vi "Main Host Json Commands.vi"(8 "error in":errorcluster, 10 "main queue":refnum<queue>, 11 "tcp in":refnum<k5>) -> (0 "error out":errorcluster, 2 "processed?":bool, 3 "tcp out":refnum<k5>)   [LabVIEW 2019]
uses:
  <vilib>/Utility/error.llb/DialogType.ctl
  RT Controls/Main Command Events.ctl
  RT Controls/Main Process Commands.ctl
panel:
  out "full cmd":string
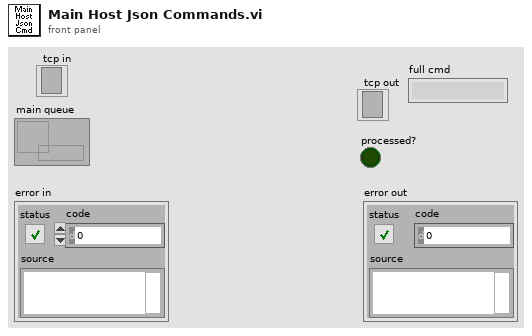
[diagram p1: front panel]
types:
  T1 = enum16{"Standard", "Buffered", "CRLF", "Immediate"}
  T2 = typedef "DialogType.ctl" = u16
  T3 = typedef "Main Process Commands.ctl" = cluster{"Commands":T4, "Value":variant}
  T4 = typedef "Main Command Events.ctl" = enum16{"Idle", "FullStop", "MainReadConfig", "MainWriteConfig", "OpenUpper", "CloseUpper", "OpenLower", "CloseLower", "SetWatchdogInt", "EnRainShutDn", "DisRainShutDn", "EnCloudShutDn", "DisCloudShutDn", "SetRainDelay", "SetLowerTimLim", "EnAutoShutDn", "DisAutoShutDn", "SetRevDelay", "RotToAz", "RotLeft", "RotRight", "RotToHome", "DefineHomePos", "SetCoast", "SetHSThres", "SetEncCounts", "SyncClose", "SyncOpen", "SetAZTimLim", "SetHomeEncPos", "SetAZTol", "SetDoorMoveTO", "AZEncPositive", "AZEncNegative", "SetShutdown", "RotToCenter"}
  T5 = cluster{"reply":string, "value":string, "error":errorcluster}
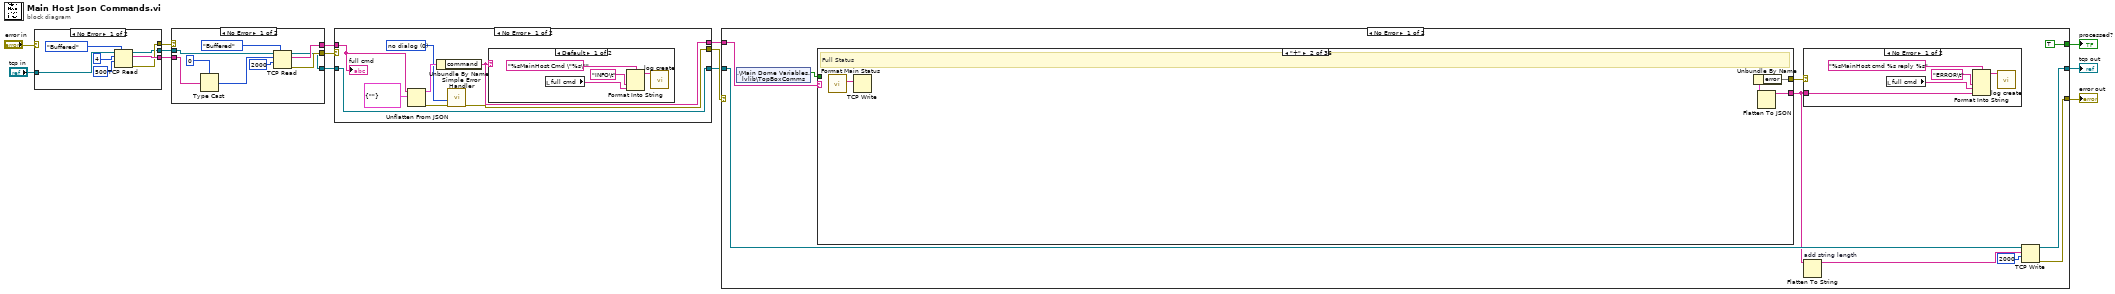
[diagram p0: block diagram]
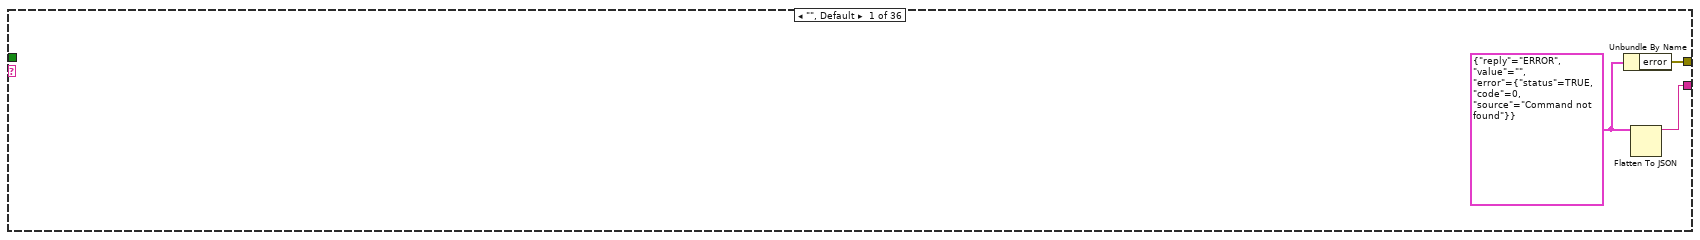
[diagram p3: hidden frame]
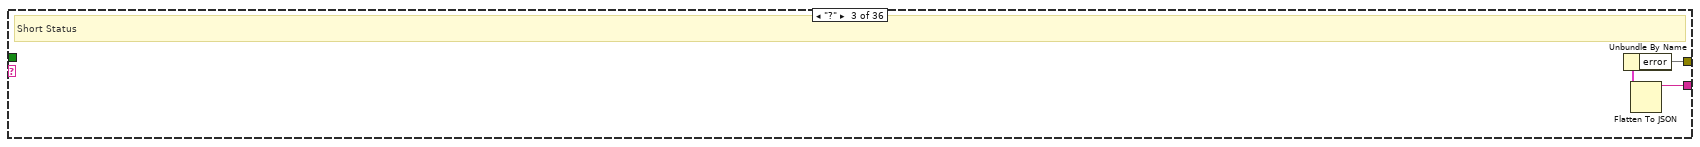
[diagram p4: hidden frame]
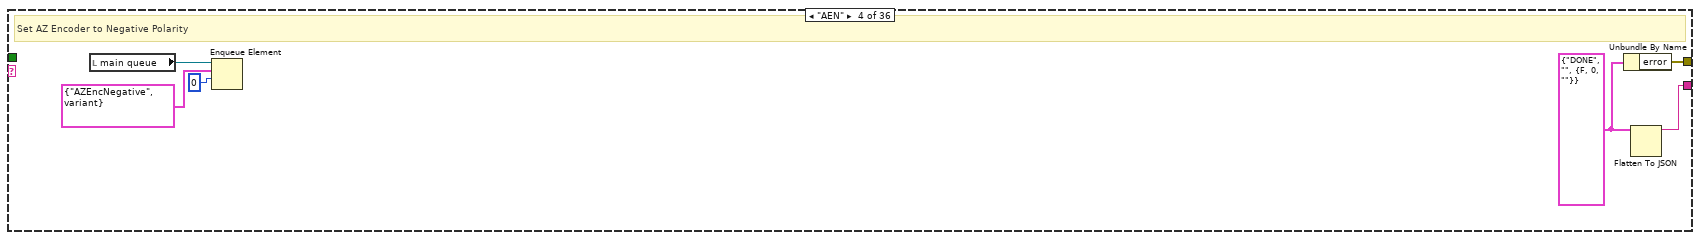
[diagram p5: hidden frame]
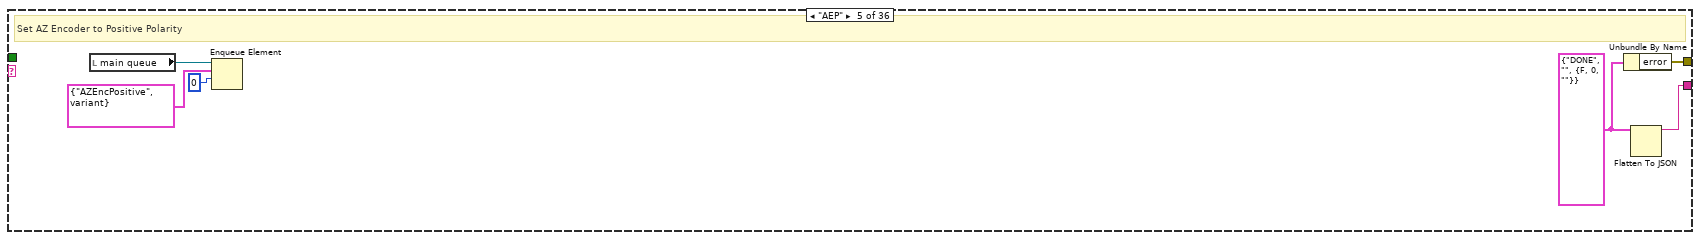
[diagram p6: hidden frame]
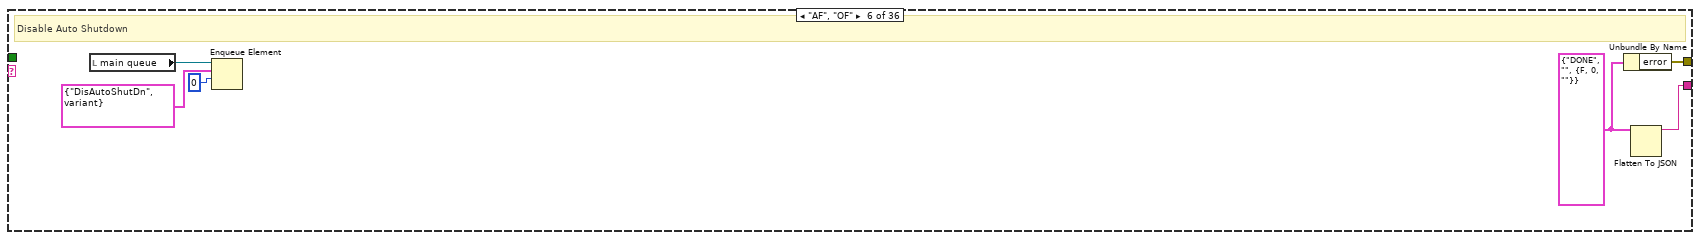
[diagram p7: hidden frame]
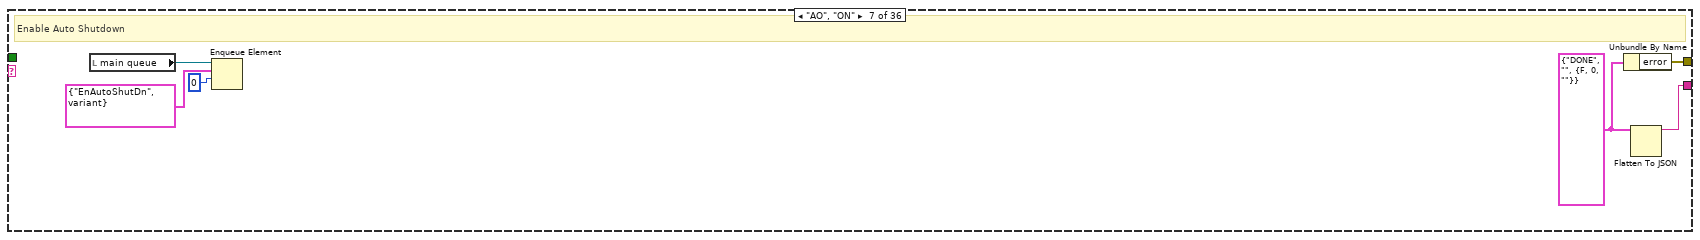
[diagram p8: hidden frame]
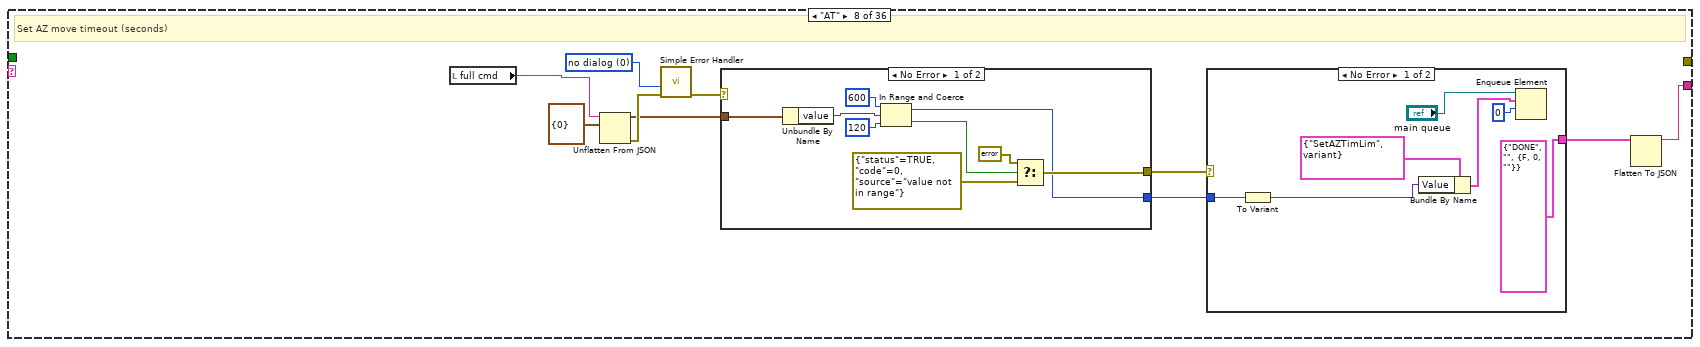
[diagram p9: hidden frame]
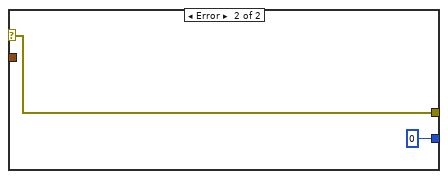
[diagram p10: hidden frame]
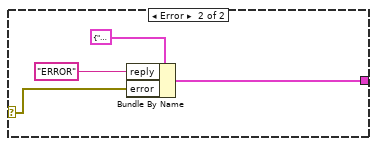
[diagram p11: hidden frame]
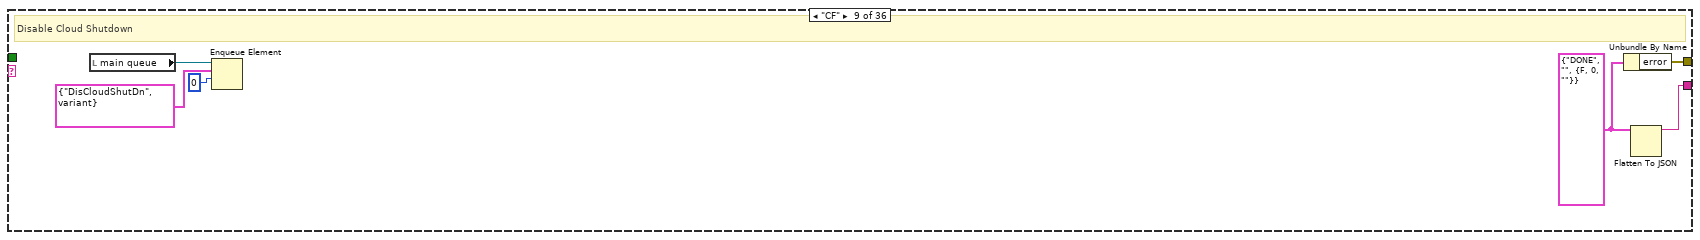
[diagram p12: hidden frame]
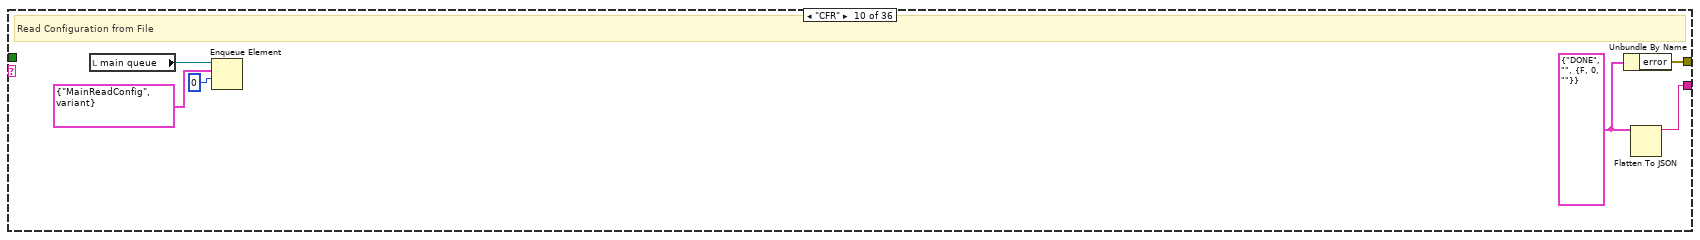
[diagram p13: hidden frame]
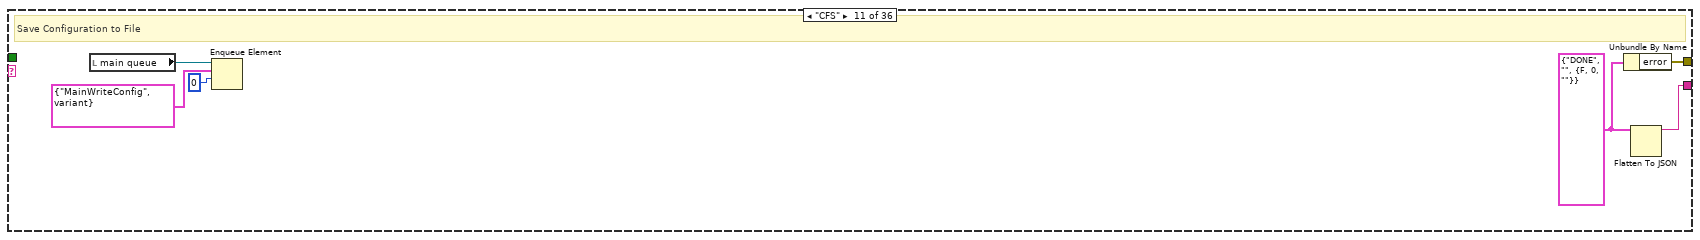
[diagram p14: hidden frame]
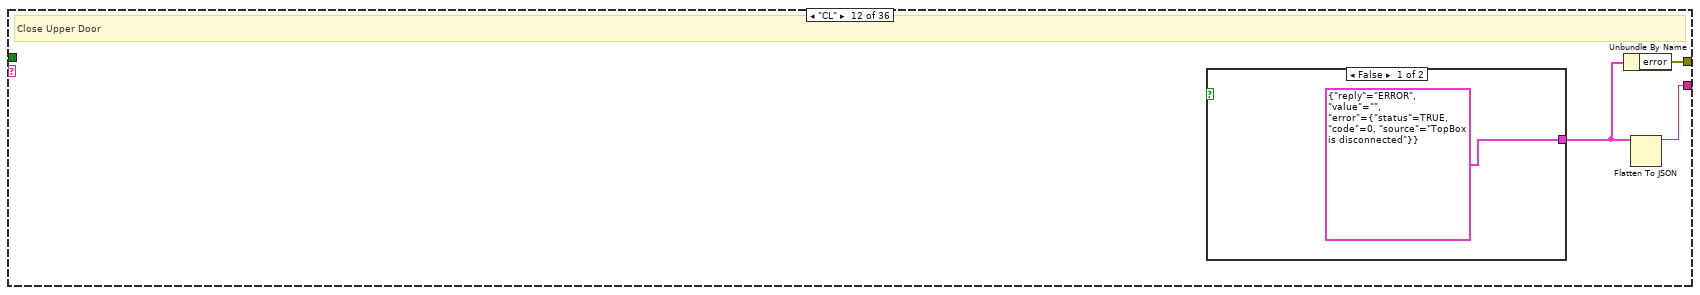
[diagram p15: hidden frame]
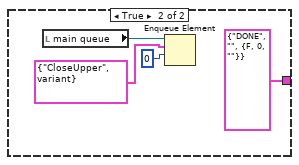
[diagram p16: hidden frame]
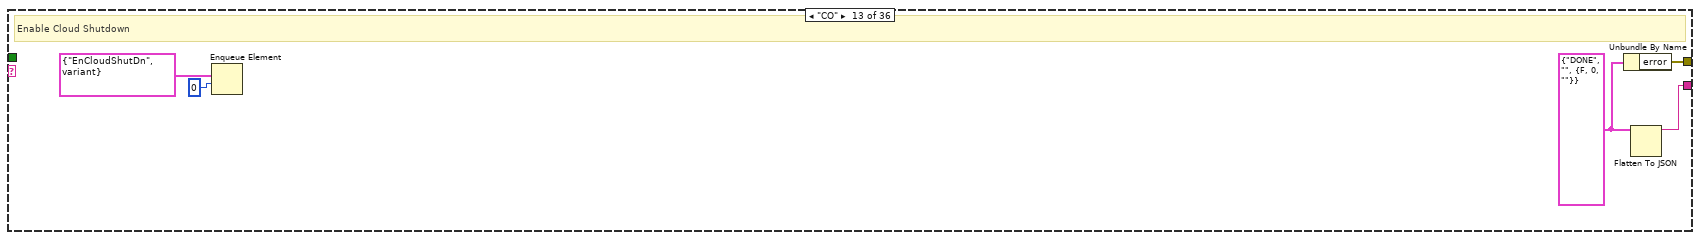
[diagram p17: hidden frame]
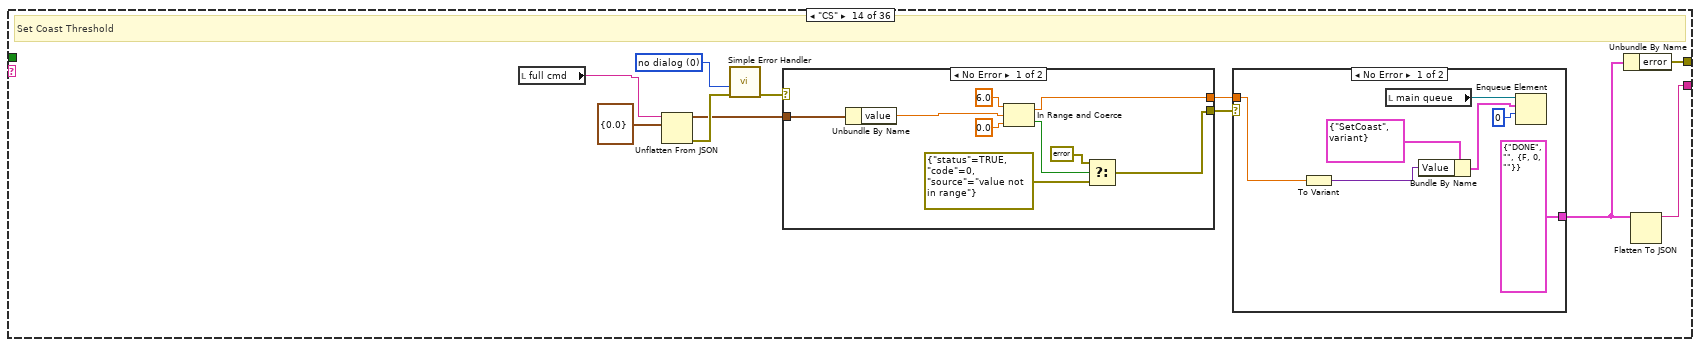
[diagram p18: hidden frame]
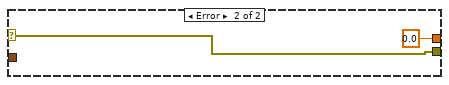
[diagram p19: hidden frame]
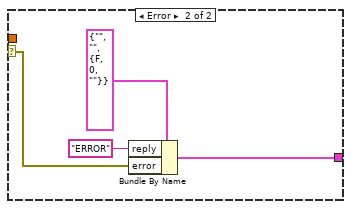
[diagram p20: hidden frame]
diagram:
  n1 = case shown="No Error" "error in" {
    selector: "error in" -> [_ w24]
    tunnel: "tcp in" -> [w21 w22]
    tunnel: [w17 "" ("data out")] -> w12
    tunnel: [w16 w24] -> w11
    tunnel: [w15 w22] -> w10
    frame No Error {
      n2 = TCP Read(connection ID=w21, bytes to read=4, 7:T1."Buffered" ("mode (standard)"), 9:500 ("timeout ms (25000)")) -> (connection ID out=w15:refnum<k5>, data out=w17:string, error out=w16:errorcluster)  [unwired: 1 in]
    }
    frame Error {
    }
  }
  n3 = case shown="No Error" w11 {
    selector: w11 -> [_ w34]
    tunnel: w12 -> [w33 _]
    tunnel: w10 -> [w31 w36]
    tunnel: [w28 w34] -> w9
    tunnel: [w27 "" ("data out")] -> w8
    tunnel: [w25 w36] -> w7
    frame No Error {
      n4 = Type Cast(type=0 ("length"), x=w33) -> (*(type *) &x=w30:i32)
      n5 = TCP Read(connection ID=w31, bytes to read=w30, 7:T1."Buffered" ("mode (standard)"), 9:2000 ("timeout ms (25000)")) -> (connection ID out=w25:refnum<k5>, data out=w27:string, error out=w28:errorcluster)  [unwired: 1 in]
    }
    frame Error {
    }
  }
  n6 = case shown="No Error" w9 {
    selector: w9 -> [_ w52]
    tunnel: w8 -> [w44 _]
    tunnel: w7 -> [w38 w51]
    tunnel: [w38 w51] -> w4
    tunnel: [w39 w50] -> w6
    tunnel: [w37 "" ("command")] -> w5
    frame No Error {
      w40 = T2 0 items=["no dialog", "OK message", "continue or stop message", "OK message + warnings", "continue/stop + warnings"] ("type of dialog (OK msg:1)")
      n7 = Unflatten From JSON(JSON string=w44, type and defaults=cluster{"command":string} {"command"=""}) -> (value=w42:cluster{"command":string}, error out=w41:errorcluster)  [unwired: 5 in]
      n8 = Unbundle By Name(w42) -> ("command"=w37:string)
      n9 = call <vilib>:"Simple Error Handler.vi"("type of dialog (OK msg:1)"=w40, "error in (no error)"=w41) -> ("error out"=w39:errorcluster)  [unwired: 3 in, 4 out]
      n10 = case shown="Default" w37 {
        frame Default {
          n11 = local read "full cmd"() -> (w45:string)
          n12 = Format Into String(format string="%sMainHost Cmd \"%s\"", "INFO\t" ("input 1"), w45) -> (resulting string=w46:string)  [unwired: 2 in, 1 out]
          n13 = call "log create.vi"("message"=w46) -> ()  [unwired: 11 in]
        }
        frame "+", "?", "HELP" {
        }
      }
      "full cmd" <- w44
    }
    frame Error {
      n14 = call <vilib>:"Clear Errors.vi"("error in (no error)"=w52, "specific error code to clear (0: all)"=56) -> ("error out"=w50:errorcluster)  [unwired: 4 in, 1 out]
    }
  }
  n15 = case shown="No Error" w6 {
    selector: w6 -> [_ w636]
    tunnel: w5 -> [w63 _]
    tunnel: w4 -> [w62 w634]
    tunnel: [w56 w636] -> w2
    tunnel: [TRUE FALSE] -> w3
    tunnel: [w58 w634] -> w1
    frame No Error {
      n16 = shared-variable ".\\Main Dome Variables.lvlib\\TopBoxComms"() -> (w54:bool)  [unwired: 1 in, 1 out]
      n17 = case shown="\"+\"" w63 {
        tunnel: [w71 w72 w76 w80 w87 w93 w99 w103 w137 w143 w149 w153 w162 w168 w202 w215 w248 w252 w257 w271 w304 w337 w368 w391 w416 w433 w458 w467 w484 w517 w542 w551 w560 w573 w598 w615] -> w59
        tunnel: [w69 w73 w77 w82 w86 w92 w98 _ w136 w142 w148 w155 w161 w166 w200 w216 w249 w251 w256 w272 w305 w338 w369 w392 w417 w434 w459 w468 w485 w518 w543 w552 w559 w574 w599 w616] -> w60
        tunnel: w54 -> [_ _ _ _ _ _ _ _ _ _ _ _ _ _ w199 w208 _ _ _ _ _ _ _ _ w415 _ w457 w466 _ _ w541 w550 _ _ w597 _]
        frame "", Default {
          w70 = T5 {"reply"="ERROR", "value"="", "error"={"status"=TRUE, "code"=0, "source"="Command not found"}} ("output cluster")
          n18 = Unbundle By Name(w70) -> ("error"=w69:errorcluster)
          n19 = Flatten To JSON(anything=w70) -> (JSON string=w71:string)  [unwired: 2 in, 1 out]
        }
        frame "+" {
          # "Full Status"
          n20 = call "Format Main Status.vi"() -> ("FullStat"=w75:string)  [unwired: 10 in, 1 out]
          n21 = TCP Write(data in=w75) -> ()  [unwired: 3 in, 3 out]
          n22 = Flatten To JSON() -> (anything=w74:cluster{}, JSON string=w72:string)  [unwired: 2 in, 1 out]
          n23 = Unbundle By Name(w74) -> ("error"=w73)
        }
        frame "?" {
          # "Short Status"
          n24 = Flatten To JSON() -> (anything=w78:cluster{}, JSON string=w76:string)  [unwired: 2 in, 1 out]
          n25 = Unbundle By Name(w78) -> ("error"=w77)
        }
        frame "AEN" {
          w81 = T5 {"reply"="DONE", "value"="", "error"={"status"=FALSE, "code"=0, "source"=""}} ("output cluster")
          # "Set AZ Encoder to Negative Polarity"
          n26 = local read "main queue"() -> (w79:refnum<queue>)
          n27 = Enqueue Element(queue=w79, element=T3 {"Commands"=enum."AZEncNegative", "Value"=variant} ("event data"), timeout in ms (-1)=0) -> ()  [unwired: 1 in, 3 out]
          n28 = Unbundle By Name(w81) -> ("error"=w82:errorcluster)
          n29 = Flatten To JSON(anything=w81) -> (JSON string=w80:string)  [unwired: 2 in, 1 out]
        }
        frame "AEP" {
          w88 = T5 {"reply"="DONE", "value"="", "error"={"status"=FALSE, "code"=0, "source"=""}} ("output cluster")
          # "Set AZ Encoder to Positive Polarity"
          n30 = local read "main queue"() -> (w85:refnum<queue>)
          n31 = Enqueue Element(queue=w85, element=T3 {"Commands"=enum."AZEncPositive", "Value"=variant} ("event data"), timeout in ms (-1)=0) -> ()  [unwired: 1 in, 3 out]
          n32 = Unbundle By Name(w88) -> ("error"=w86:errorcluster)
          n33 = Flatten To JSON(anything=w88) -> (JSON string=w87:string)  [unwired: 2 in, 1 out]
        }
        frame "AF", "OF" {
          w94 = T5 {"reply"="DONE", "value"="", "error"={"status"=FALSE, "code"=0, "source"=""}} ("output cluster")
          # "Disable Auto Shutdown"
          n34 = local read "main queue"() -> (w91:refnum<queue>)
          n35 = Enqueue Element(queue=w91, element=T3 {"Commands"=enum."DisAutoShutDn", "Value"=variant} ("event data"), timeout in ms (-1)=0) -> ()  [unwired: 1 in, 3 out]
          n36 = Unbundle By Name(w94) -> ("error"=w92:errorcluster)
          n37 = Flatten To JSON(anything=w94) -> (JSON string=w93:string)  [unwired: 2 in, 1 out]
        }
        frame "AO", "ON" {
          w100 = T5 {"reply"="DONE", "value"="", "error"={"status"=FALSE, "code"=0, "source"=""}} ("output cluster")
          # "Enable Auto Shutdown"
          n38 = local read "main queue"() -> (w97:refnum<queue>)
          n39 = Enqueue Element(queue=w97, element=T3 {"Commands"=enum."EnAutoShutDn", "Value"=variant} ("event data"), timeout in ms (-1)=0) -> ()  [unwired: 1 in, 3 out]
          n40 = Unbundle By Name(w100) -> ("error"=w98:errorcluster)
          n41 = Flatten To JSON(anything=w100) -> (JSON string=w99:string)  [unwired: 2 in, 1 out]
        }
        frame "AT" {
          w109 = T2 0 items=["no dialog", "OK message", "continue or stop message", "OK message + warnings", "continue/stop + warnings"] ("type of dialog (OK msg:1)")
          # "Set AZ move timeout (seconds)"
          n42 = local read "full cmd"() -> (w111:string)
          n43 = Unflatten From JSON(JSON string=w111, type and defaults=cluster{"value":i32} {"value"=0}) -> (value=w107:cluster{"value":i32}, error out=w110:errorcluster)  [unwired: 5 in]
          n44 = call <vilib>:"Simple Error Handler.vi"("type of dialog (OK msg:1)"=w109, "error in (no error)"=w110) -> ("error out"=w108:errorcluster)  [unwired: 3 in, 4 out]
          n45 = case shown="No Error" w108 {
            selector: w108 -> [_ w123]
            tunnel: w107 -> [w121 _]
            tunnel: [w115 w123] -> w106
            tunnel: [w113 0 ("upper limit")] -> w105
            frame No Error {
              n46 = Unbundle By Name(w121) -> ("value"=w118:i32)
              n47 = In Range and Coerce(upper limit=600, x=w118, lower limit=120) -> (coerced(x)=w113:i32, In Range?=w117:bool)
              n48 = Select(t=errorcluster {"status"=FALSE, "code"=0, "source"=""} ("error IO"), s=w117, f=errorcluster {"status"=TRUE, "code"=0, "source"="value not in range"}) -> (s? t:f=w115:errorcluster)
            }
            frame Error {
            }
          }
          n49 = case shown="No Error" w106 {
            selector: w106 -> [_ w133]
            tunnel: w105 -> [w130 _]
            tunnel: [T5 {"reply"="DONE", "value"="", "error"={"status"=FALSE, "code"=0, "source"=""}} ("output cluster") w132] -> w104
            frame No Error {
              n50 = To Variant(anything=w130) -> (Variant=w129:variant)
              n51 = Bundle By Name(cluster=T3 {"Commands"=enum."SetAZTimLim", "Value"=variant} ("event data"), "Value"=w129) -> (w126:T3)
              n52 = Enqueue Element(queue="main queue", element=w126, timeout in ms (-1)=0) -> ()  [unwired: 1 in, 3 out]
            }
            frame Error {
              n53 = Bundle By Name(cluster=T5 {"reply"="", "value"="", "error"={"status"=FALSE, "code"=0, "source"=""}} ("output cluster"), "reply"="ERROR", "error"=w133) -> (w132:T5)
            }
          }
          n54 = Flatten To JSON(anything=w104) -> (JSON string=w103:string)  [unwired: 2 in, 1 out]
        }
        frame "CF" {
          w138 = T5 {"reply"="DONE", "value"="", "error"={"status"=FALSE, "code"=0, "source"=""}} ("output cluster")
          # "Disable Cloud Shutdown"
          n55 = local read "main queue"() -> (w135:refnum<queue>)
          n56 = Enqueue Element(queue=w135, element=T3 {"Commands"=enum."DisCloudShutDn", "Value"=variant} ("event data"), timeout in ms (-1)=0) -> ()  [unwired: 1 in, 3 out]
          n57 = Unbundle By Name(w138) -> ("error"=w136:errorcluster)
          n58 = Flatten To JSON(anything=w138) -> (JSON string=w137:string)  [unwired: 2 in, 1 out]
        }
        frame "CFR" {
          w144 = T5 {"reply"="DONE", "value"="", "error"={"status"=FALSE, "code"=0, "source"=""}} ("output cluster")
          # "Read Configuration from File"
          n59 = local read "main queue"() -> (w141:refnum<queue>)
          n60 = Enqueue Element(queue=w141, element=T3 {"Commands"=enum."MainReadConfig", "Value"=variant} ("event data"), timeout in ms (-1)=0) -> ()  [unwired: 1 in, 3 out]
          n61 = Unbundle By Name(w144) -> ("error"=w142:errorcluster)
          n62 = Flatten To JSON(anything=w144) -> (JSON string=w143:string)  [unwired: 2 in, 1 out]
        }
        frame "CFS" {
          w150 = T5 {"reply"="DONE", "value"="", "error"={"status"=FALSE, "code"=0, "source"=""}} ("output cluster")
          # "Save Configuration to File"
          n63 = local read "main queue"() -> (w147:refnum<queue>)
          n64 = Enqueue Element(queue=w147, element=T3 {"Commands"=enum."MainWriteConfig", "Value"=variant} ("event data"), timeout in ms (-1)=0) -> ()  [unwired: 1 in, 3 out]
          n65 = Unbundle By Name(w150) -> ("error"=w148:errorcluster)
          n66 = Flatten To JSON(anything=w150) -> (JSON string=w149:string)  [unwired: 2 in, 1 out]
        }
        frame "CL" {
          # "Close Upper Door"
          n67 = case shown="False" {
            selector: _ -> [_ _]
            tunnel: [T5 {"reply"="ERROR", "value"="", "error"={"status"=TRUE, "code"=0, "source"="TopBox is disconnected"}} ("output cluster") T5 {"reply"="DONE", "value"="", "error"={"status"=FALSE, "code"=0, "source"=""}} ("output cluster")] -> w154
            frame False {
            }
            frame True {
              n68 = local read "main queue"() -> (w158:refnum<queue>)
              n69 = Enqueue Element(queue=w158, element=T3 {"Commands"=enum."CloseUpper", "Value"=variant} ("event data"), timeout in ms (-1)=0) -> ()  [unwired: 1 in, 3 out]
            }
          }
          n70 = Unbundle By Name(w154) -> ("error"=w155:errorcluster)
          n71 = Flatten To JSON(anything=w154) -> (JSON string=w153:string)  [unwired: 2 in, 1 out]
        }
        frame "CO" {
          w163 = T5 {"reply"="DONE", "value"="", "error"={"status"=FALSE, "code"=0, "source"=""}} ("output cluster")
          # "Enable Cloud Shutdown"
          n72 = Enqueue Element(element=T3 {"Commands"=enum."EnCloudShutDn", "Value"=variant} ("event data"), timeout in ms (-1)=0) -> ()  [unwired: 2 in, 3 out]
          n73 = Unbundle By Name(w163) -> ("error"=w161:errorcluster)
          n74 = Flatten To JSON(anything=w163) -> (JSON string=w162:string)  [unwired: 2 in, 1 out]
        }
        frame "CS" {
          w174 = T2 0 items=["no dialog", "OK message", "continue or stop message", "OK message + warnings", "continue/stop + warnings"] ("type of dialog (OK msg:1)")
          # "Set Coast Threshold"
          n75 = local read "full cmd"() -> (w173:string)
          n76 = Unflatten From JSON(JSON string=w173, type and defaults=cluster{"value":dbl} {"value"=0.0}) -> (value=w171:cluster{"value":dbl}, error out=w175:errorcluster)  [unwired: 5 in]
          n77 = call <vilib>:"Simple Error Handler.vi"("type of dialog (OK msg:1)"=w174, "error in (no error)"=w175) -> ("error out"=w172:errorcluster)  [unwired: 3 in, 4 out]
          n78 = case shown="No Error" w172 {
            selector: w172 -> [_ w187]
            tunnel: [w179 w187] -> w169
            tunnel: w171 -> [w183 _]
            tunnel: [w177 0.0 ("upper limit")] -> w170
            frame No Error {
              n79 = Unbundle By Name(w183) -> ("value"=w182:dbl)
              n80 = In Range and Coerce(upper limit=6.0, x=w182, lower limit=0.0) -> (coerced(x)=w177:dbl, In Range?=w181:bool)
              n81 = Select(t=errorcluster {"status"=FALSE, "code"=0, "source"=""} ("error IO"), s=w181, f=errorcluster {"status"=TRUE, "code"=0, "source"="value not in range"}) -> (s? t:f=w179:errorcluster)
            }
            frame Error {
            }
          }
          n82 = case shown="No Error" w169 {
            selector: w169 -> [_ w196]
            tunnel: w170 -> [w194 _]
            tunnel: [T5 {"reply"="DONE", "value"="", "error"={"status"=FALSE, "code"=0, "source"=""}} ("output cluster") w195] -> w167
            frame No Error {
              n83 = To Variant(anything=w194) -> (Variant=w193:variant)
              n84 = local read "main queue"() -> (w189:refnum<queue>)
              n85 = Bundle By Name(cluster=T3 {"Commands"=enum."SetCoast", "Value"=variant} ("event data"), "Value"=w193) -> (w190:T3)
              n86 = Enqueue Element(queue=w189, element=w190, timeout in ms (-1)=0) -> ()  [unwired: 1 in, 3 out]
            }
            frame Error {
              n87 = Bundle By Name(cluster=T5 {"reply"="", "value"="", "error"={"status"=FALSE, "code"=0, "source"=""}} ("output cluster"), "reply"="ERROR", "error"=w196) -> (w195:T5)
            }
          }
          n88 = Unbundle By Name(w167) -> ("error"=w166:errorcluster)
          n89 = Flatten To JSON(anything=w167) -> (JSON string=w168:string)  [unwired: 2 in, 1 out]
        }
        frame "DN" {
          # "Open Lower Door"
          n90 = case shown="True" w199 {
            tunnel: [T5 {"reply"="ERROR", "value"="", "error"={"status"=TRUE, "code"=0, "source"="TopBox is disconnected"}} ("output cluster") T5 {"reply"="DONE", "value"="", "error"={"status"=FALSE, "code"=0, "source"=""}} ("output cluster")] -> w201
            frame False {
            }
            frame True {
              n91 = local read "main queue"() -> (w204:refnum<queue>)
              n92 = Enqueue Element(queue=w204, element=T3 {"Commands"=enum."OpenLower", "Value"=variant} ("event data"), timeout in ms (-1)=0) -> ()  [unwired: 1 in, 3 out]
            }
          }
          n93 = Unbundle By Name(w201) -> ("error"=w200:errorcluster)
          n94 = Flatten To JSON(anything=w201) -> (JSON string=w202:string)  [unwired: 2 in, 1 out]
        }
        frame "DT" {
          # "Set Door Move Timeout (sec)"
          n95 = case shown="True" w208 {
            tunnel: [w246 errorcluster {"status"=FALSE, "code"=0, "source"=""} ("error")] -> w214
            frame False {
              w246 = errorcluster {"status"=TRUE, "code"=0, "source"="TopBox is disconnected"}  # error
            }
            frame True {
            }
          }
          n96 = case shown="No Error" w214 {
            selector: w214 -> [_ w245]
            tunnel: [w239 w245] -> w213
            tunnel: [w237 0.0 ("value")] -> w212
            frame No Error {
              w241 = T2 0 items=["no dialog", "OK message", "continue or stop message", "OK message + warnings", "continue/stop + warnings"] ("type of dialog (OK msg:1)")
              n97 = local read "full cmd"() -> (w240:string)
              n98 = Unflatten From JSON(JSON string=w240, type and defaults=cluster{"value":dbl} {"value"=0.0}) -> (value=w238:cluster{"value":dbl}, error out=w242:errorcluster)  [unwired: 5 in]
              n99 = Unbundle By Name(w238) -> ("value"=w237:dbl)
              n100 = call <vilib>:"Simple Error Handler.vi"("type of dialog (OK msg:1)"=w241, "error in (no error)"=w242) -> ("error out"=w239:errorcluster)  [unwired: 3 in, 4 out]
            }
            frame Error {
            }
          }
          n101 = case shown="No Error" w213 {
            selector: w213 -> [_ w236]
            tunnel: w212 -> [w231 _]
            tunnel: [w232 0.0 ("upper limit")] -> w211
            tunnel: [w228 w236] -> w210
            frame No Error {
              n102 = In Range and Coerce(upper limit=600.0, x=w231, lower limit=30.0) -> (coerced(x)=w232:dbl, In Range?=w230:bool)
              n103 = Select(t=errorcluster {"status"=FALSE, "code"=0, "source"=""} ("error IO"), s=w230, f=errorcluster {"status"=TRUE, "code"=0, "source"="value out of range"}) -> (s? t:f=w228:errorcluster)
            }
            frame Error {
            }
          }
          n104 = case shown="No Error" w210 {
            selector: w210 -> [_ w225]
            tunnel: w211 -> [w222 _]
            tunnel: [T5 {"reply"="DONE", "value"="", "error"={"status"=FALSE, "code"=0, "source"=""}} ("output cluster") w223] -> w209
            frame No Error {
              n105 = To Variant(anything=w222) -> (Variant=w221:variant)
              n106 = Bundle By Name(cluster=T3 {"Commands"=enum."SetDoorMoveTO", "Value"=variant} ("event data"), "Value"=w221) -> (w218:T3)
              n107 = Enqueue Element(element=w218, timeout in ms (-1)=0) -> ()  [unwired: 2 in, 3 out]
            }
            frame Error {
              n108 = Bundle By Name(cluster=T5 {"reply"="", "value"="", "error"={"status"=FALSE, "code"=0, "source"=""}} ("output cluster"), "reply"="ERROR", "error"=w225) -> (w223:T5)
            }
          }
          n109 = Unbundle By Name(w209) -> ("error"=w216:errorcluster)
          n110 = Flatten To JSON(anything=w209) -> (JSON string=w215:string)  [unwired: 2 in, 1 out]
        }
        frame "HELP" {
          # "Help"
          n111 = Flatten To JSON() -> (anything=w250:cluster{}, JSON string=w248:string)  [unwired: 2 in, 1 out]
          n112 = Unbundle By Name(w250) -> ("error"=w249)
        }
        frame "HM" {
          w253 = T5 {"reply"="DONE", "value"="", "error"={"status"=FALSE, "code"=0, "source"=""}} ("output cluster")
          # "Send Dome to Home"
          n113 = Enqueue Element(element=T3 {"Commands"=enum."RotToHome", "Value"=variant} ("event data"), timeout in ms (-1)=0) -> ()  [unwired: 2 in, 3 out]
          n114 = Unbundle By Name(w253) -> ("error"=w251:errorcluster)
          n115 = Flatten To JSON(anything=w253) -> (JSON string=w252:string)  [unwired: 2 in, 1 out]
        }
        frame "CN" {
          w258 = T5 {"reply"="DONE", "value"="", "error"={"status"=FALSE, "code"=0, "source"=""}} ("output cluster")
          # "Send Dome to Center"
          n116 = Enqueue Element(element=T3 {"Commands"=enum."RotToCenter", "Value"=variant} ("event data"), timeout in ms (-1)=0) -> ()  [unwired: 2 in, 3 out]
          n117 = Unbundle By Name(w258) -> ("error"=w256:errorcluster)
          n118 = Flatten To JSON(anything=w258) -> (JSON string=w257:string)  [unwired: 2 in, 1 out]
        }
        frame "HS" {
          w267 = T2 0 items=["no dialog", "OK message", "continue or stop message", "OK message + warnings", "continue/stop + warnings"] ("type of dialog (OK msg:1)")
          # "Set High Speed Threshold (deg)"
          n119 = local read "full cmd"() -> (w269:string)
          n120 = Unflatten From JSON(JSON string=w269, type and defaults=cluster{"value":dbl} {"value"=0.0}) -> (value=w268:cluster{"value":dbl}, error out=w270:errorcluster)  [unwired: 5 in]
          n121 = Unbundle By Name(w268) -> ("value"=w264:dbl)
          n122 = call <vilib>:"Simple Error Handler.vi"("type of dialog (OK msg:1)"=w267, "error in (no error)"=w270) -> ("error out"=w265:errorcluster)  [unwired: 3 in, 4 out]
          n123 = case shown="No Error" w265 {
            selector: w265 -> [_ w282]
            tunnel: w264 -> [w278 _]
            tunnel: [w277 0.0 ("upper limit")] -> w263
            tunnel: [w273 w282] -> w262
            frame No Error {
              n124 = In Range and Coerce(upper limit=10.0, x=w278, lower limit=0.0) -> (coerced(x)=w277:dbl, In Range?=w276:bool)
              n125 = Select(t=errorcluster {"status"=FALSE, "code"=0, "source"=""} ("error IO"), s=w276, f=errorcluster {"status"=TRUE, "code"=0, "source"="value out of range"}) -> (s? t:f=w273:errorcluster)
            }
            frame Error {
            }
          }
          n126 = case shown="Error .." w262 {
            selector: w262 -> [_ w292]
            tunnel: w263 -> [w289 _]
            tunnel: [T5 {"reply"="DONE", "value"="", "error"={"status"=FALSE, "code"=0, "source"=""}} ("output cluster") w290] -> w261
            frame No Error {
              n127 = To Variant(anything=w289) -> (Variant=w288:variant)
              n128 = local read "main queue"() -> (w284:refnum<queue>)
              n129 = Bundle By Name(cluster=T3 {"Commands"=enum."SetHSThres", "Value"=variant} ("event data"), "Value"=w288) -> (w285:T3)
              n130 = Enqueue Element(queue=w284, element=w285, timeout in ms (-1)=0) -> ()  [unwired: 1 in, 3 out]
            }
            frame Error {
              n131 = Bundle By Name(cluster=T5 {"reply"="", "value"="", "error"={"status"=FALSE, "code"=0, "source"=""}} ("output cluster"), "reply"="ERROR", "error"=w292) -> (w290:T5)
            }
          }
          n132 = Unbundle By Name(w261) -> ("error"=w272:errorcluster)
          n133 = Flatten To JSON(anything=w261) -> (JSON string=w271:string)  [unwired: 2 in, 1 out]
        }
        frame "HZ" {
          w298 = T2 0 items=["no dialog", "OK message", "continue or stop message", "OK message + warnings", "continue/stop + warnings"] ("type of dialog (OK msg:1)")
          # "Define Dome Home Position (degs)"
          n134 = local read "full cmd"() -> (w302:string)
          n135 = Unflatten From JSON(JSON string=w302, type and defaults=cluster{"value":dbl} {"value"=0.0}) -> (value=w301:cluster{"value":dbl}, error out=w303:errorcluster)  [unwired: 5 in]
          n136 = Unbundle By Name(w301) -> ("value"=w299:dbl)
          n137 = call <vilib>:"Simple Error Handler.vi"("type of dialog (OK msg:1)"=w298, "error in (no error)"=w303) -> ("error out"=w300:errorcluster)  [unwired: 3 in, 4 out]
          n138 = case shown="No Error" w300 {
            selector: w300 -> [_ w315]
            tunnel: w299 -> [w311 _]
            tunnel: [w310 0.0 ("upper limit")] -> w296
            tunnel: [w306 w315] -> w295
            frame No Error {
              n139 = In Range and Coerce(upper limit=360.0, x=w311, lower limit=0.0) -> (coerced(x)=w310:dbl, In Range?=w309:bool)
              n140 = Select(t=errorcluster {"status"=FALSE, "code"=0, "source"=""} ("error IO"), s=w309, f=errorcluster {"status"=TRUE, "code"=0, "source"="value out of range"}) -> (s? t:f=w306:errorcluster)
            }
            frame Error {
            }
          }
          n141 = case shown="No Error" w295 {
            selector: w295 -> [_ w323]
            tunnel: w296 -> [w322 _]
            tunnel: [T5 {"reply"="DONE", "value"="", "error"={"status"=FALSE, "code"=0, "source"=""}} ("output cluster") w324] -> w294
            frame No Error {
              n142 = To Variant(anything=w322) -> (Variant=w321:variant)
              n143 = local read "main queue"() -> (w316:refnum<queue>)
              n144 = Bundle By Name(cluster=T3 {"Commands"=enum."DefineHomePos", "Value"=variant} ("event data"), "Value"=w321) -> (w318:T3)
              n145 = Enqueue Element(queue=w316, element=w318, timeout in ms (-1)=0) -> ()  [unwired: 1 in, 3 out]
            }
            frame Error {
              n146 = Bundle By Name(cluster=T5 {"reply"="", "value"="", "error"={"status"=FALSE, "code"=0, "source"=""}} ("output cluster"), "reply"="ERROR", "error"=w323) -> (w324:T5)
            }
          }
          n147 = Unbundle By Name(w294) -> ("error"=w305:errorcluster)
          n148 = Flatten To JSON(anything=w294) -> (JSON string=w304:string)  [unwired: 2 in, 1 out]
        }
        frame "LF" {
          w329 = T2 0 items=["no dialog", "OK message", "continue or stop message", "OK message + warnings", "continue/stop + warnings"] ("type of dialog (OK msg:1)")
          # "Rotate Dome Left by Degrees"
          n149 = local read "full cmd"() -> (w335:string)
          n150 = Unflatten From JSON(JSON string=w335, type and defaults=cluster{"value":dbl} {"value"=0.0}) -> (value=w334:cluster{"value":dbl}, error out=w336:errorcluster)  [unwired: 5 in]
          n151 = Unbundle By Name(w334) -> ("value"=w332:dbl)
          n152 = call <vilib>:"Simple Error Handler.vi"("type of dialog (OK msg:1)"=w329, "error in (no error)"=w336) -> ("error out"=w333:errorcluster)  [unwired: 3 in, 4 out]
          n153 = case shown="No Error" w333 {
            selector: w333 -> [_ w348]
            tunnel: w332 -> [w344 _]
            tunnel: [w343 0.0 ("upper limit")] -> w331
            tunnel: [w339 w348] -> w330
            frame No Error {
              n154 = In Range and Coerce(upper limit=360.0, x=w344, lower limit=0.0) -> (coerced(x)=w343:dbl, In Range?=w342:bool)
              n155 = Select(t=errorcluster {"status"=FALSE, "code"=0, "source"=""} ("error IO"), s=w342, f=errorcluster {"status"=TRUE, "code"=0, "source"="value out of range"}) -> (s? t:f=w339:errorcluster)
            }
            frame Error {
            }
          }
          n156 = case shown="No Error" w330 {
            selector: w330 -> [_ w356]
            tunnel: w331 -> [w355 _]
            tunnel: [T5 {"reply"="DONE", "value"="", "error"={"status"=FALSE, "code"=0, "source"=""}} ("output cluster") w357] -> w327
            frame No Error {
              n157 = To Variant(anything=w355) -> (Variant=w354:variant)
              n158 = local read "main queue"() -> (w349:refnum<queue>)
              n159 = Bundle By Name(cluster=T3 {"Commands"=enum."RotLeft", "Value"=variant} ("event data"), "Value"=w354) -> (w351:T3)
              n160 = Enqueue Element(queue=w349, element=w351, timeout in ms (-1)=0) -> ()  [unwired: 1 in, 3 out]
            }
            frame Error {
              n161 = Bundle By Name(cluster=T5 {"reply"="", "value"="", "error"={"status"=FALSE, "code"=0, "source"=""}} ("output cluster"), "reply"="ERROR", "error"=w356) -> (w357:T5)
            }
          }
          n162 = Unbundle By Name(w327) -> ("error"=w338:errorcluster)
          n163 = Flatten To JSON(anything=w327) -> (JSON string=w337:string)  [unwired: 2 in, 1 out]
        }
        frame "LM" {
          w364 = T2 0 items=["no dialog", "OK message", "continue or stop message", "OK message + warnings", "continue/stop + warnings"] ("type of dialog (OK msg:1)")
          # "Encoder Counts in 360 degrees"
          n164 = local read "full cmd"() -> (w366:string)
          n165 = Unflatten From JSON(JSON string=w366, type and defaults=cluster{"value":u64} {"value"=0}) -> (value=w365:cluster{"value":u64}, error out=w367:errorcluster)  [unwired: 5 in]
          n166 = Unbundle By Name(w365) -> ("value"=w361:u64)
          n167 = call <vilib>:"Simple Error Handler.vi"("type of dialog (OK msg:1)"=w364, "error in (no error)"=w367) -> ("error out"=w362:errorcluster)  [unwired: 3 in, 4 out]
          n168 = case shown="No Error" w362 {
            selector: w362 -> [_ w377]
            tunnel: w361 -> [w376 _]
            tunnel: [T5 {"reply"="DONE", "value"="", "error"={"status"=FALSE, "code"=0, "source"=""}} ("output cluster") w378] -> w360
            frame No Error {
              n169 = To Variant(anything=w376) -> (Variant=w375:variant)
              n170 = local read "main queue"() -> (w370:refnum<queue>)
              n171 = Bundle By Name(cluster=T3 {"Commands"=enum."SetEncCounts", "Value"=variant} ("event data"), "Value"=w375) -> (w372:T3)
              n172 = Enqueue Element(queue=w370, element=w372, timeout in ms (-1)=0) -> ()  [unwired: 1 in, 3 out]
            }
            frame Error {
              n173 = Bundle By Name(cluster=T5 {"reply"="", "value"="", "error"={"status"=FALSE, "code"=0, "source"=""}} ("output cluster"), "reply"="ERROR", "error"=w377) -> (w378:T5)
            }
          }
          n174 = Unbundle By Name(w360) -> ("error"=w369:errorcluster)
          n175 = Flatten To JSON(anything=w360) -> (JSON string=w368:string)  [unwired: 2 in, 1 out]
        }
        frame "MV" {
          w383 = T2 0 items=["no dialog", "OK message", "continue or stop message", "OK message + warnings", "continue/stop + warnings"] ("type of dialog (OK msg:1)")
          # "Rotate Dome to Az Position (deg)"
          n176 = local read "full cmd"() -> (w389:string)
          n177 = Unflatten From JSON(JSON string=w389, type and defaults=cluster{"value":dbl} {"value"=0.0}) -> (value=w388:cluster{"value":dbl}, error out=w390:errorcluster)  [unwired: 5 in]
          n178 = Unbundle By Name(w388) -> ("value"=w386:dbl)
          n179 = call <vilib>:"Simple Error Handler.vi"("type of dialog (OK msg:1)"=w383, "error in (no error)"=w390) -> ("error out"=w387:errorcluster)  [unwired: 3 in, 4 out]
          n180 = case shown="No Error" w387 {
            selector: w387 -> [_ w402]
            tunnel: w386 -> [w398 _]
            tunnel: [w397 0.0 ("upper limit")] -> w385
            tunnel: [w393 w402] -> w384
            frame No Error {
              n181 = In Range and Coerce(upper limit=360.0, x=w398, lower limit=0.0) -> (coerced(x)=w397:dbl, In Range?=w396:bool)
              n182 = Select(t=errorcluster {"status"=FALSE, "code"=0, "source"=""} ("error IO"), s=w396, f=errorcluster {"status"=TRUE, "code"=0, "source"="value out of range"}) -> (s? t:f=w393:errorcluster)
            }
            frame Error {
            }
          }
          n183 = case shown="No Error" w384 {
            selector: w384 -> [_ w410]
            tunnel: w385 -> [w409 _]
            tunnel: [T5 {"reply"="DONE", "value"="", "error"={"status"=FALSE, "code"=0, "source"=""}} ("output cluster") w411] -> w381
            frame No Error {
              n184 = To Variant(anything=w409) -> (Variant=w408:variant)
              n185 = local read "main queue"() -> (w403:refnum<queue>)
              n186 = Bundle By Name(cluster=T3 {"Commands"=enum."RotToAz", "Value"=variant} ("event data"), "Value"=w408) -> (w405:T3)
              n187 = Enqueue Element(queue=w403, element=w405, timeout in ms (-1)=0) -> ()  [unwired: 1 in, 3 out]
            }
            frame Error {
              n188 = Bundle By Name(cluster=T5 {"reply"="", "value"="", "error"={"status"=FALSE, "code"=0, "source"=""}} ("output cluster"), "reply"="ERROR", "error"=w410) -> (w411:T5)
            }
          }
          n189 = Unbundle By Name(w381) -> ("error"=w392:errorcluster)
          n190 = Flatten To JSON(anything=w381) -> (JSON string=w391:string)  [unwired: 2 in, 1 out]
        }
        frame "OP" {
          # "Open Upper Door"
          n191 = case shown="False" w415 {
            tunnel: [T5 {"reply"="ERROR", "value"="", "error"={"status"=TRUE, "code"=0, "source"="TopBox is disconnected"}} ("output cluster") T5 {"reply"="DONE", "value"="", "error"={"status"=FALSE, "code"=0, "source"=""}} ("output cluster")] -> w414
            frame False {
            }
            frame True {
              n192 = local read "main queue"() -> (w419:refnum<queue>)
              n193 = Enqueue Element(queue=w419, element=T3 {"Commands"=enum."OpenUpper", "Value"=variant} ("event data"), timeout in ms (-1)=0) -> ()  [unwired: 1 in, 3 out]
            }
          }
          n194 = Unbundle By Name(w414) -> ("error"=w417:errorcluster)
          n195 = Flatten To JSON(anything=w414) -> (JSON string=w416:string)  [unwired: 2 in, 1 out]
        }
        frame "RD" {
          w425 = T2 0 items=["no dialog", "OK message", "continue or stop message", "OK message + warnings", "continue/stop + warnings"] ("type of dialog (OK msg:1)")
          # "Set Reverse Direction Delay (s)"
          n196 = local read "full cmd"() -> (w431:string)
          n197 = Unflatten From JSON(JSON string=w431, type and defaults=cluster{"value":i32} {"value"=0}) -> (value=w430:cluster{"value":i32}, error out=w432:errorcluster)  [unwired: 5 in]
          n198 = Unbundle By Name(w430) -> ("value"=w428:i32)
          n199 = call <vilib>:"Simple Error Handler.vi"("type of dialog (OK msg:1)"=w425, "error in (no error)"=w432) -> ("error out"=w429:errorcluster)  [unwired: 3 in, 4 out]
          n200 = case shown="No Error" w429 {
            selector: w429 -> [_ w444]
            tunnel: w428 -> [w440 _]
            tunnel: [w439 0 ("upper limit")] -> w427
            tunnel: [w435 w444] -> w426
            frame No Error {
              n201 = In Range and Coerce(upper limit=6, x=w440, lower limit=0) -> (coerced(x)=w439:i32, In Range?=w438:bool)
              n202 = Select(t=errorcluster {"status"=FALSE, "code"=0, "source"=""} ("error IO"), s=w438, f=errorcluster {"status"=TRUE, "code"=0, "source"="value out of range"}) -> (s? t:f=w435:errorcluster)
            }
            frame Error {
            }
          }
          n203 = case shown="No Error" w426 {
            selector: w426 -> [_ w452]
            tunnel: w427 -> [w451 _]
            tunnel: [T5 {"reply"="DONE", "value"="", "error"={"status"=FALSE, "code"=0, "source"=""}} ("output cluster") w453] -> w423
            frame No Error {
              n204 = To Variant(anything=w451) -> (Variant=w450:variant)
              n205 = local read "main queue"() -> (w445:refnum<queue>)
              n206 = Bundle By Name(cluster=T3 {"Commands"=enum."SetRevDelay", "Value"=variant} ("event data"), "Value"=w450) -> (w447:T3)
              n207 = Enqueue Element(queue=w445, element=w447, timeout in ms (-1)=0) -> ()  [unwired: 1 in, 3 out]
            }
            frame Error {
              n208 = Bundle By Name(cluster=T5 {"reply"="", "value"="", "error"={"status"=FALSE, "code"=0, "source"=""}} ("output cluster"), "reply"="ERROR", "error"=w452) -> (w453:T5)
            }
          }
          n209 = Unbundle By Name(w423) -> ("error"=w434:errorcluster)
          n210 = Flatten To JSON(anything=w423) -> (JSON string=w433:string)  [unwired: 2 in, 1 out]
        }
        frame "RF" {
          # "Disable Rail-Snow Shutdown"
          n211 = case shown="True" w457 {
            tunnel: [T5 {"reply"="ERROR", "value"="", "error"={"status"=TRUE, "code"=0, "source"="TopBox is disconnected"}} ("output cluster") T5 {"reply"="DONE", "value"="", "error"={"status"=FALSE, "code"=0, "source"=""}} ("output cluster")] -> w456
            frame False {
            }
            frame True {
              n212 = local read "main queue"() -> (w462:refnum<queue>)
              n213 = Enqueue Element(queue=w462, element=T3 {"Commands"=enum."DisRainShutDn", "Value"=variant} ("event data"), timeout in ms (-1)=0) -> ()  [unwired: 1 in, 3 out]
            }
          }
          n214 = Unbundle By Name(w456) -> ("error"=w459:errorcluster)
          n215 = Flatten To JSON(anything=w456) -> (JSON string=w458:string)  [unwired: 2 in, 1 out]
        }
        frame "RO" {
          # "Enable Rain-Snow Shutdown"
          n216 = case shown="True" w466 {
            tunnel: [T5 {"reply"="ERROR", "value"="", "error"={"status"=TRUE, "code"=0, "source"="TopBox is disconnected"}} ("output cluster") T5 {"reply"="DONE", "value"="", "error"={"status"=FALSE, "code"=0, "source"=""}} ("output cluster")] -> w465
            frame False {
            }
            frame True {
              n217 = local read "main queue"() -> (w471:refnum<queue>)
              n218 = Enqueue Element(queue=w471, element=T3 {"Commands"=enum."EnRainShutDn", "Value"=variant} ("event data"), timeout in ms (-1)=0) -> ()  [unwired: 1 in, 3 out]
            }
          }
          n219 = Unbundle By Name(w465) -> ("error"=w468:errorcluster)
          n220 = Flatten To JSON(anything=w465) -> (JSON string=w467:string)  [unwired: 2 in, 1 out]
        }
        frame "RS" {
          w476 = T2 0 items=["no dialog", "OK message", "continue or stop message", "OK message + warnings", "continue/stop + warnings"] ("type of dialog (OK msg:1)")
          # "Set Rain/Snow Activate Delay"
          n221 = local read "full cmd"() -> (w482:string)
          n222 = Unflatten From JSON(JSON string=w482, type and defaults=cluster{"value":i32} {"value"=0}) -> (value=w481:cluster{"value":i32}, error out=w483:errorcluster)  [unwired: 5 in]
          n223 = Unbundle By Name(w481) -> ("value"=w479:i32)
          n224 = call <vilib>:"Simple Error Handler.vi"("type of dialog (OK msg:1)"=w476, "error in (no error)"=w483) -> ("error out"=w480:errorcluster)  [unwired: 3 in, 4 out]
          n225 = case shown="No Error" w480 {
            selector: w480 -> [_ w495]
            tunnel: w479 -> [w491 _]
            tunnel: [w490 0 ("upper limit")] -> w478
            tunnel: [w486 w495] -> w477
            frame No Error {
              n226 = In Range and Coerce(upper limit=10, x=w491, lower limit=1) -> (coerced(x)=w490:i32, In Range?=w489:bool)
              n227 = Select(t=errorcluster {"status"=FALSE, "code"=0, "source"=""} ("error IO"), s=w489, f=errorcluster {"status"=TRUE, "code"=0, "source"="value out of range"}) -> (s? t:f=w486:errorcluster)
            }
            frame Error {
            }
          }
          n228 = case shown="No Error" w477 {
            selector: w477 -> [_ w503]
            tunnel: w478 -> [w502 _]
            tunnel: [T5 {"reply"="DONE", "value"="", "error"={"status"=FALSE, "code"=0, "source"=""}} ("output cluster") w504] -> w474
            frame No Error {
              n229 = To Variant(anything=w502) -> (Variant=w501:variant)
              n230 = local read "main queue"() -> (w496:refnum<queue>)
              n231 = Bundle By Name(cluster=T3 {"Commands"=enum."SetRainDelay", "Value"=variant} ("event data"), "Value"=w501) -> (w498:T3)
              n232 = Enqueue Element(queue=w496, element=w498, timeout in ms (-1)=0) -> ()  [unwired: 1 in, 3 out]
            }
            frame Error {
              n233 = Bundle By Name(cluster=T5 {"reply"="", "value"="", "error"={"status"=FALSE, "code"=0, "source"=""}} ("output cluster"), "reply"="ERROR", "error"=w503) -> (w504:T5)
            }
          }
          n234 = Unbundle By Name(w474) -> ("error"=w485:errorcluster)
          n235 = Flatten To JSON(anything=w474) -> (JSON string=w484:string)  [unwired: 2 in, 1 out]
        }
        frame "RT" {
          w509 = T2 0 items=["no dialog", "OK message", "continue or stop message", "OK message + warnings", "continue/stop + warnings"] ("type of dialog (OK msg:1)")
          # "Rotate Dome Right by Degrees"
          n236 = local read "full cmd"() -> (w515:string)
          n237 = Unflatten From JSON(JSON string=w515, type and defaults=cluster{"value":dbl} {"value"=0.0}) -> (value=w514:cluster{"value":dbl}, error out=w516:errorcluster)  [unwired: 5 in]
          n238 = Unbundle By Name(w514) -> ("value"=w512:dbl)
          n239 = call <vilib>:"Simple Error Handler.vi"("type of dialog (OK msg:1)"=w509, "error in (no error)"=w516) -> ("error out"=w513:errorcluster)  [unwired: 3 in, 4 out]
          n240 = case shown="No Error" w513 {
            selector: w513 -> [_ w528]
            tunnel: w512 -> [w524 _]
            tunnel: [w523 0.0 ("upper limit")] -> w511
            tunnel: [w519 w528] -> w510
            frame No Error {
              n241 = In Range and Coerce(upper limit=360.0, x=w524, lower limit=0.0) -> (coerced(x)=w523:dbl, In Range?=w522:bool)
              n242 = Select(t=errorcluster {"status"=FALSE, "code"=0, "source"=""} ("error IO"), s=w522, f=errorcluster {"status"=TRUE, "code"=0, "source"="value out of range"}) -> (s? t:f=w519:errorcluster)
            }
            frame Error {
            }
          }
          n243 = case shown="No Error" w510 {
            selector: w510 -> [_ w536]
            tunnel: w511 -> [w535 _]
            tunnel: [T5 {"reply"="DONE", "value"="", "error"={"status"=FALSE, "code"=0, "source"=""}} ("output cluster") w537] -> w507
            frame No Error {
              n244 = To Variant(anything=w535) -> (Variant=w534:variant)
              n245 = local read "main queue"() -> (w529:refnum<queue>)
              n246 = Bundle By Name(cluster=T3 {"Commands"=enum."RotRight", "Value"=variant} ("event data"), "Value"=w534) -> (w531:T3)
              n247 = Enqueue Element(queue=w529, element=w531, timeout in ms (-1)=0) -> ()  [unwired: 1 in, 3 out]
            }
            frame Error {
              n248 = Bundle By Name(cluster=T5 {"reply"="", "value"="", "error"={"status"=FALSE, "code"=0, "source"=""}} ("output cluster"), "reply"="ERROR", "error"=w536) -> (w537:T5)
            }
          }
          n249 = Unbundle By Name(w507) -> ("error"=w518:errorcluster)
          n250 = Flatten To JSON(anything=w507) -> (JSON string=w517:string)  [unwired: 2 in, 1 out]
        }
        frame "SC" {
          # "Sync Close"
          n251 = case shown="True" w541 {
            tunnel: [T5 {"reply"="ERROR", "value"="", "error"={"status"=TRUE, "code"=0, "source"="TopBox is disconnected"}} ("output cluster") T5 {"reply"="DONE", "value"="", "error"={"status"=FALSE, "code"=0, "source"=""}} ("output cluster")] -> w540
            frame False {
            }
            frame True {
              n252 = local read "main queue"() -> (w546:refnum<queue>)
              n253 = Enqueue Element(queue=w546, element=T3 {"Commands"=enum."SyncClose", "Value"=variant} ("event data"), timeout in ms (-1)=0) -> ()  [unwired: 1 in, 3 out]
            }
          }
          n254 = Unbundle By Name(w540) -> ("error"=w543:errorcluster)
          n255 = Flatten To JSON(anything=w540) -> (JSON string=w542:string)  [unwired: 2 in, 1 out]
        }
        frame "SO" {
          # "Sync Open"
          n256 = case shown="True" w550 {
            tunnel: [T5 {"reply"="ERROR", "value"="", "error"={"status"=TRUE, "code"=0, "source"="TopBox is disconnected"}} ("output cluster") T5 {"reply"="DONE", "value"="", "error"={"status"=FALSE, "code"=0, "source"=""}} ("output cluster")] -> w549
            frame False {
            }
            frame True {
              n257 = local read "main queue"() -> (w555:refnum<queue>)
              n258 = Enqueue Element(queue=w555, element=T3 {"Commands"=enum."SyncOpen", "Value"=variant} ("event data"), timeout in ms (-1)=0) -> ()  [unwired: 1 in, 3 out]
            }
          }
          n259 = Unbundle By Name(w549) -> ("error"=w552:errorcluster)
          n260 = Flatten To JSON(anything=w549) -> (JSON string=w551:string)  [unwired: 2 in, 1 out]
        }
        frame "ST" {
          w561 = T5 {"reply"="DONE", "value"="", "error"={"status"=FALSE, "code"=0, "source"=""}} ("output cluster")
          # "Full Stop"
          n261 = local read "main queue"() -> (w558:refnum<queue>)
          n262 = Lossy Enqueue Element(queue=w558, element=T3 {"Commands"=enum."FullStop", "Value"=variant} ("event data")) -> ()  [unwired: 1 in, 4 out]
          n263 = Unbundle By Name(w561) -> ("error"=w559:errorcluster)
          n264 = Flatten To JSON(anything=w561) -> (JSON string=w560:string)  [unwired: 2 in, 1 out]
        }
        frame "TOL" {
          w565 = T2 0 items=["no dialog", "OK message", "continue or stop message", "OK message + warnings", "continue/stop + warnings"] ("type of dialog (OK msg:1)")
          # "Set AZ Position Tolerance (deg)"
          n265 = local read "full cmd"() -> (w571:string)
          n266 = Unflatten From JSON(JSON string=w571, type and defaults=cluster{"value":dbl} {"value"=0.0}) -> (value=w570:cluster{"value":dbl}, error out=w572:errorcluster)  [unwired: 5 in]
          n267 = Unbundle By Name(w570) -> ("value"=w568:dbl)
          n268 = call <vilib>:"Simple Error Handler.vi"("type of dialog (OK msg:1)"=w565, "error in (no error)"=w572) -> ("error out"=w569:errorcluster)  [unwired: 3 in, 4 out]
          n269 = case shown="No Error" w569 {
            selector: w569 -> [_ w584]
            tunnel: w568 -> [w580 _]
            tunnel: [w579 0.0 ("upper limit")] -> w567
            tunnel: [w575 w584] -> w566
            frame No Error {
              n270 = In Range and Coerce(upper limit=3.0, x=w580, lower limit=0.0) -> (coerced(x)=w579:dbl, In Range?=w578:bool)
              n271 = Select(t=errorcluster {"status"=FALSE, "code"=0, "source"=""} ("error IO"), s=w578, f=errorcluster {"status"=TRUE, "code"=0, "source"="value out of range"}) -> (s? t:f=w575:errorcluster)
            }
            frame Error {
            }
          }
          n272 = case shown="Error .." w566 {
            selector: w566 -> [_ w592]
            tunnel: w567 -> [w591 _]
            tunnel: [T5 {"reply"="DONE", "value"="", "error"={"status"=FALSE, "code"=0, "source"=""}} ("output cluster") w593] -> w563
            frame No Error {
              n273 = To Variant(anything=w591) -> (Variant=w590:variant)
              n274 = local read "main queue"() -> (w585:refnum<queue>)
              n275 = Bundle By Name(cluster=T3 {"Commands"=enum."SetAZTol", "Value"=variant} ("event data"), "Value"=w590) -> (w587:T3)
              n276 = Enqueue Element(queue=w585, element=w587, timeout in ms (-1)=0) -> ()  [unwired: 1 in, 3 out]
            }
            frame Error {
              n277 = Bundle By Name(cluster=T5 {"reply"="", "value"="", "error"={"status"=FALSE, "code"=0, "source"=""}} ("output cluster"), "reply"="ERROR", "error"=w592) -> (w593:T5)
            }
          }
          n278 = Unbundle By Name(w563) -> ("error"=w574:errorcluster)
          n279 = Flatten To JSON(anything=w563) -> (JSON string=w573:string)  [unwired: 2 in, 1 out]
        }
        frame "UP" {
          # "Close Lower Door"
          n280 = case shown="True" w597 {
            tunnel: [T5 {"reply"="ERROR", "value"="", "error"={"status"=TRUE, "code"=0, "source"="TopBox is disconnected"}} ("output cluster") T5 {"reply"="DONE", "value"="", "error"={"status"=FALSE, "code"=0, "source"=""}} ("output cluster")] -> w596
            frame False {
            }
            frame True {
              n281 = local read "main queue"() -> (w602:refnum<queue>)
              n282 = Enqueue Element(queue=w602, element=T3 {"Commands"=enum."CloseLower", "Value"=variant} ("event data"), timeout in ms (-1)=0) -> ()  [unwired: 1 in, 3 out]
            }
          }
          n283 = Unbundle By Name(w596) -> ("error"=w599:errorcluster)
          n284 = Flatten To JSON(anything=w596) -> (JSON string=w598:string)  [unwired: 2 in, 1 out]
        }
        frame "WT" {
          w611 = T2 0 items=["no dialog", "OK message", "continue or stop message", "OK message + warnings", "continue/stop + warnings"] ("type of dialog (OK msg:1)")
          # "Set Watchdog Timer Interval"
          n285 = local read "full cmd"() -> (w613:string)
          n286 = Unflatten From JSON(JSON string=w613, type and defaults=cluster{"value":i32} {"value"=0}) -> (value=w612:cluster{"value":i32}, error out=w614:errorcluster)  [unwired: 5 in]
          n287 = Unbundle By Name(w612) -> ("value"=w608:i32)
          n288 = call <vilib>:"Simple Error Handler.vi"("type of dialog (OK msg:1)"=w611, "error in (no error)"=w614) -> ("error out"=w609:errorcluster)  [unwired: 3 in, 4 out]
          n289 = case shown="No Error" w609 {
            selector: w609 -> [_ w622]
            tunnel: w608 -> [w617 _]
            tunnel: [w618 w622] -> w606
            tunnel: [w617 _] -> w607
            frame No Error {
              n290 = Greater Than 0?(x=w617) -> (x > 0?=w621:bool)
              n291 = Select(t=errorcluster {"status"=FALSE, "code"=0, "source"=""} ("error IO"), s=w621, f=errorcluster {"status"=TRUE, "code"=0, "source"="value out of range"}) -> (s? t:f=w618:errorcluster)
            }
            frame Error {
            }
          }
          n292 = case shown="Error .." w606 {
            selector: w606 -> [_ w632]
            tunnel: w607 -> [w628 _]
            tunnel: [T5 {"reply"="DONE", "value"="", "error"={"status"=FALSE, "code"=0, "source"=""}} ("output cluster") w630] -> w605
            frame No Error {
              n293 = To Variant(anything=w628) -> (Variant=w627:variant)
              n294 = local read "main queue"() -> (w624:refnum<queue>)
              n295 = Bundle By Name(cluster=T3 {"Commands"=enum."SetWatchdogInt", "Value"=variant} ("event data"), "Value"=w627) -> (w625:T3)
              n296 = Enqueue Element(queue=w624, element=w625, timeout in ms (-1)=0) -> ()  [unwired: 1 in, 3 out]
            }
            frame Error {
              n297 = Bundle By Name(cluster=T5 {"reply"="", "value"="", "error"={"status"=FALSE, "code"=0, "source"=""}} ("output cluster"), "reply"="ERROR", "error"=w632) -> (w630:T5)
            }
          }
          n298 = Unbundle By Name(w605) -> ("error"=w616:errorcluster)
          n299 = Flatten To JSON(anything=w605) -> (JSON string=w615:string)  [unwired: 2 in, 1 out]
        }
      }
      n300 = case shown="No Error" w60 {
        tunnel: w59 -> [w64 _]
        frame No Error {
          n301 = local read "full cmd"() -> (w65:string)
          n302 = Format Into String(format string="%sMainHost cmd %s reply %s", "ERROR\t" ("input 1"), w65, w64) -> (resulting string=w67:string)  [unwired: 2 in, 1 out]
          n303 = call "log create.vi"("message"=w67) -> ()  [unwired: 11 in]
        }
        frame Error {
        }
      }
      n304 = Flatten To String "add string length"(anything=w59) -> (data string=w61:string)  [unwired: 3 in, 2 out]
      n305 = TCP Write(connection ID=w62, data in=w61, 9:2000 ("timeout ms (25000)")) -> (connection ID out=w58:refnum<k5>, error out=w56:errorcluster)  [unwired: 1 in, 1 out]
    }
    frame Error {
    }
  }
  "error out" <- w2
  "tcp out" <- w1
  "processed?" <- w3
